vi "Hindbrain Main.vi"(9 "Boat Type":T1(ring), 11 "NotifierReff":T2) -> ()   [LabVIEW 2013]
uses:
  Data/TypeDefs/Notifiers.ctl
  Data/TypeDefs/UTM Location.ctl
  Data/TypeDefs/Sail Set Suggestions.ctl
  Data/TypeDefs/Rudder Set Suggestions.ctl
  <vilib>/myRIO/Common/Instrument Driver Framework/myRIO v1.0/UART/vis/myRIO v1.0 Close UART.vi
  <vilib>/myRIO/Common/Instrument Driver Framework/Utilities/vis/FPGA Ref Manager.vi
  <vilib>/myRIO/Common/Instrument Driver Framework/myRIO v1.0/myRIO v1.0 Reset FPGA.vi
  <vilib>/myRIO/Instrument Drivers/Utilities/Utilities.lvlib
panel:
  in  "XBee Serial Port":refnum<visa-resource-name>
  in  "Queue timeout (ms)":i32=200
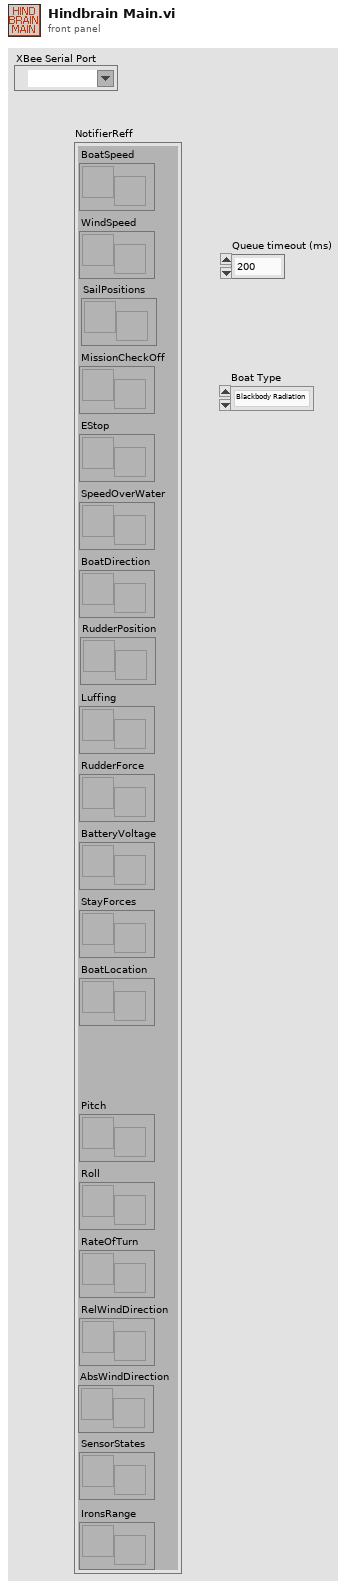
[diagram p1: front panel]
types:
  T1 = enum16{"Blackbody Radiation", "Little boats", "Simulation", "Damn Yankee"}
  T2 = typedef "Notifiers.ctl" = cluster{"BoatSpeed":refnum<notifier>, "WindSpeed":refnum<notifier>, "MissionCheckOff":refnum<notifier>, "EStop":refnum<notifier>, "SpeedOverWater":refnum<notifier>, "BoatDirection":refnum<notifier>, "Luffing":refnum<notifier>, "RudderForce":refnum<notifier>, "BatteryVoltage":refnum<notifier>, "StayForces":refnum<notifier>, "BoatLocation":refnum<notifier>, "Pitch":refnum<notifier>, "Roll":refnum<notifier>, "RateOfTurn":refnum<notifier>, "RelWindDirection":refnum<notifier>, "SailPositions":refnum<notifier>, "RudderPosition":refnum<notifier>, "SensorStates":refnum<notifier>, "IronsRange":refnum<notifier>, "AbsWindDirection":refnum<notifier>}
  T3 = typedef "UTM Location.ctl" = cluster{"UTM Zone":dbl, "Hemisphere":enum16{"North", "South"}, "East":dbl, "North":dbl}
  T4 = typedef "PWM.lvlib/PWM Reference.ctl" = cluster{"myRIO Reference":T5, "PWM Channels Enum":T9, "PWM Configuration":T10}
  T5 = typedef "myRIO Generic Hardware Reference.ctl" = cluster{"myRIO Model":T6, "myRIO Hardware Reference":T7}
  T6 = typedef "Hardware Version Enum.ctl" = enum16{"Unknown", "myRIO-1900", "myRIO-1950"}
  T7 = typedef "myRIO v1.0 Reference.ctl" = cluster{"Generic FPGA Reference":T8, "Allow multiple opens":bool}
  T8 = typedef "Generic FPGA Reference.ctl" = refnum<k20>
  T9 = typedef "PWM Channels Enum.ctl" = enum16{"Not Connected", "C/PWM0", "C/PWM1", "A/PWM0", "A/PWM1", "A/PWM2", "B/PWM0", "B/PWM1", "B/PWM2"}
  T10 = typedef "PWM.lvlib/PWM Configuration.ctl" = cluster{"Frequency":dbl, "Duty Cycle":dbl}
  T11 = cluster{"Airmar VISA Resource":refnum<visa-resource-name>, "Hemisphere VISA Resource":refnum<visa-resource-name>, "Dynamixel VISA Resource":refnum<visa-resource-name>, "Airmar Error":errorcluster, "Hemisphere Error":errorcluster, "Dynamixel Error":errorcluster, "OLD Airmar Refernce Number":refnum<visa-resource-name>, "Rudder PWM Ref":T4, "Rudder Error":errorcluster}
  T12 = typedef "GPS-Compass Queue Cluster.ctl" = cluster{"BoatLocation Queue":refnum<queue>, "BoatDirection Queue":refnum<queue>, "BoatSpeed Queue":refnum<queue>, "RateOfTurn Queue":refnum<queue>, "Pitch Queue":refnum<queue>, "Roll Queue":refnum<queue>}
  T13 = typedef "WindData Queue Cluster.ctl" = cluster{"RelWindDirection Queue":refnum<queue>, "WindSpeed Queue":refnum<queue>, "AbsWindDirection Queue":refnum<queue>}
  T14 = cluster{"Rudder Queue":refnum<queue>, "Shroud Queue":refnum<queue>, "Battery Voltage Queue":refnum<queue>, "Accelerometer Queue":refnum<queue>, "AirmarGPS-Compass Queue Cluster":T12, "Hemisphere Queue Cluster":T12, "Airmar Wind Queue Cluster":T13, "Wind Vane Queue Cluster":T13, "Little Boat Queues":cluster{"Heading Queue":refnum<queue>, "Location Queue":refnum<queue>, "Wind Speed Queue":refnum<queue>, "Tilt Queue":refnum<queue>, "Wind Direction Queue":refnum<queue>}}
  T15 = typedef "Sail Set Suggestions.ctl" = cluster{"MainSailSuggestion":dbl, "JibSailSuggestion":dbl}
  T16 = typedef "Rudder Set Suggestions.ctl" = dbl
  T17 = cluster{"AirmarOnline":bool, "WindvaneOnline":bool, "HemisphereOnline":bool, "RudderForceOnline":bool, "StayForceOnline":bool, "BatteryVoltageOnline":bool, "AccelerometerOnline":bool}
  T18 = cluster{"Nav Data":cluster{"regular expression":string, i32, i32, i32}, "Nav Data":cluster{"regular expression":string, i32, i32, i32}}
  T19 = cluster{"regular expression":string, i32, i32, i32}
  T20 = cluster{"Heading Queue":refnum<queue>, "Location Queue":refnum<queue>, "Wind Speed Queue":refnum<queue>, "Tilt Queue":refnum<queue>, "Wind Direction Queue":refnum<queue>}
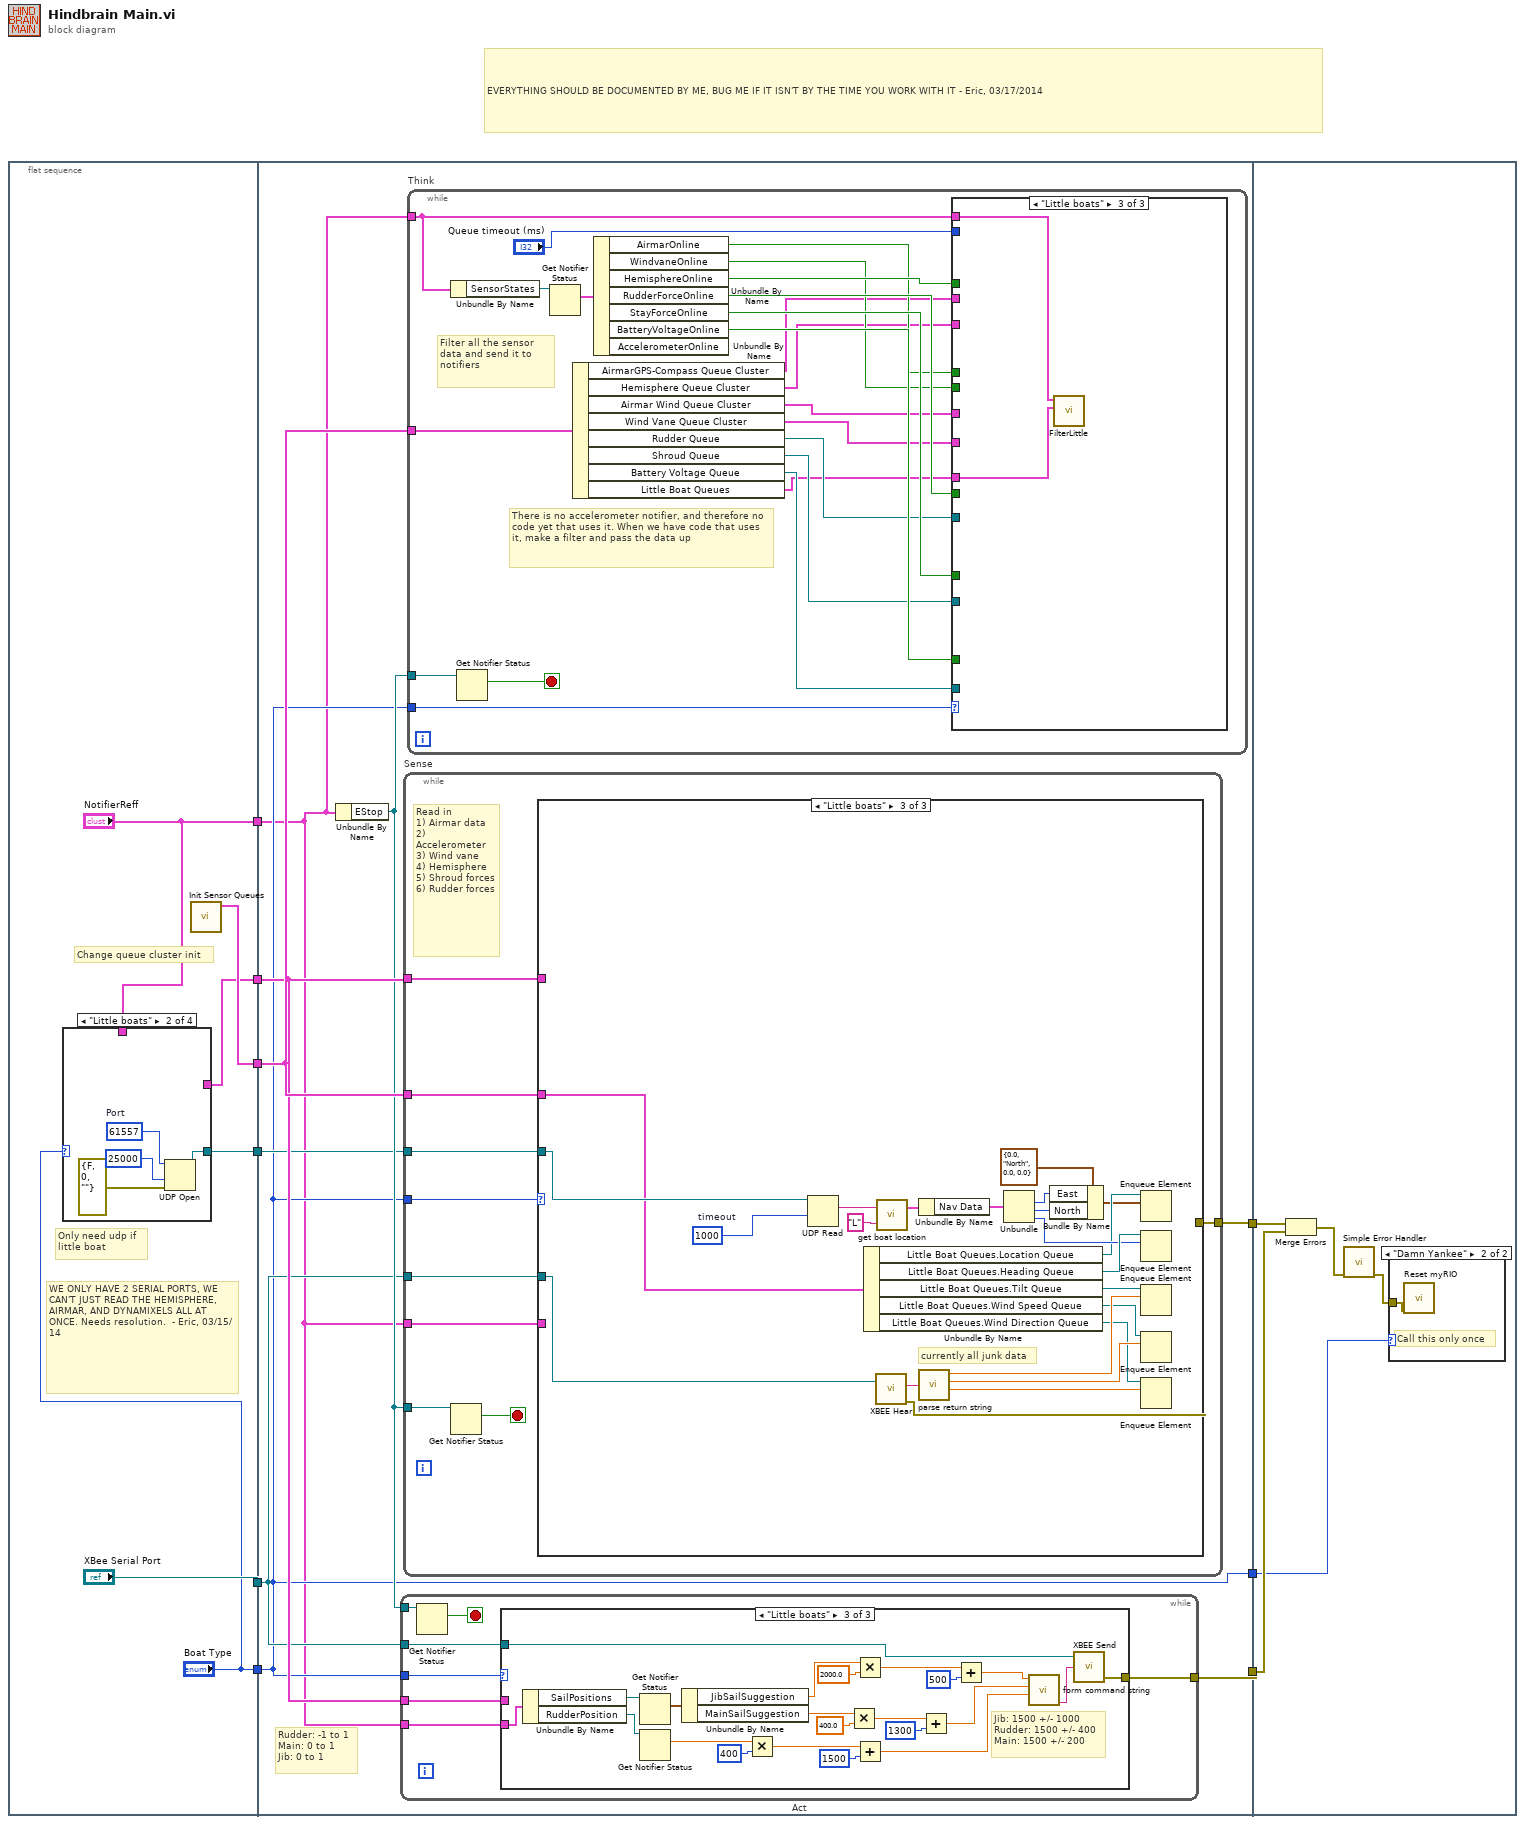
[diagram p0: block diagram]
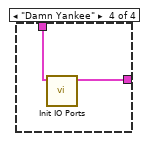
[diagram p4: hidden frame]
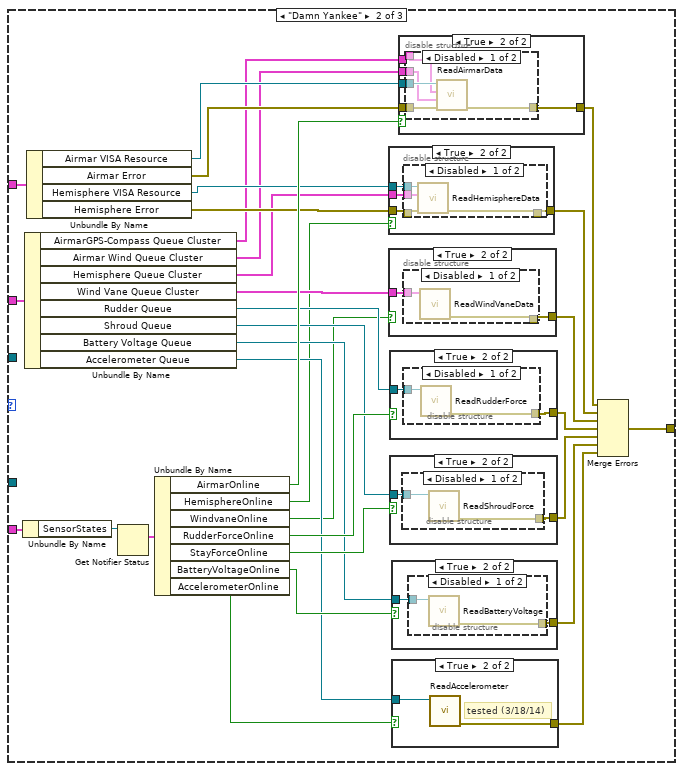
[diagram p6: hidden frame]
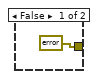
[diagram p7: hidden frame]
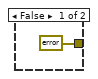
[diagram p8: hidden frame]
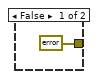
[diagram p10: hidden frame]
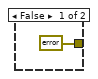
[diagram p12: hidden frame]
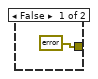
[diagram p14: hidden frame]
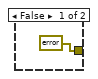
[diagram p16: hidden frame]
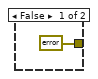
[diagram p18: hidden frame]
diagram:
  # "EVERYTHING SHOULD BE DOCUMENTED BY ME, BUG ME IF IT ISN'T BY THE TIME YOU WORK WITH IT - Eric, 03/17/2014"
  n1 = flat-sequence {
    tunnel: [w15] -> w7
    tunnel: [w11] -> w6
    tunnel: ["Boat Type"] -> w5
    tunnel: ["XBee Serial Port"] -> w4
    tunnel: [w13] -> w3
    tunnel: ["NotifierReff"] -> w1
    tunnel: [w30] -> w9
    tunnel: [w29] -> w8
    tunnel: w7 -> [w28]
    tunnel: w6 -> [w27]
    tunnel: w5 -> [w23]
    tunnel: w4 -> [w25]
    tunnel: w3 -> [w24]
    tunnel: [w23] -> w2
    tunnel: w1 -> [w22]
    tunnel: w9 -> [w255]
    tunnel: w8 -> [w256]
    tunnel: w2 -> [w254]
    frame #0 {
      # "Only need udp if\nlittle boat"
      # "Change queue cluster init"
      # "WE ONLY HAVE 2 SERIAL PORTS, WE CAN'T JUST READ THE HEMISPHERE, AIRMAR, AND DYNAMIXELS ALL AT ONCE. Needs resolution.  - Eric, 03/15/14"
      n2 = case shown="\"Little boats\"" "Boat Type" {
        tunnel: [_ w16 _ _] -> w13
        tunnel: [_ _ _ w21] -> w11
        tunnel: "NotifierReff" -> [_ _ _ w20]
        frame "Blackbody Radiation", Default {
        }
        frame "Little boats" {
          w18 = u16 61557  # Port
          n3 = UDP Open(8:errorcluster {"status"=FALSE, "code"=0, "source"=""} ("error in (no error)"), 9:25000 ("timeout ms (25000)"), 11:w18) -> (port=w16:refnum<k16>)  [unwired: 2 in, 2 out]
        }
        frame "Simulation" {
        }
        frame "Damn Yankee" {
          n4 = call "Init IO Ports.vi"("NotifierReff"=w20) -> ("IO Port Cluster"=w21:T11)  [unwired: 10 in]
        }
      }
      n5 = call "Init Sensor Queues.vi"() -> ("Hindbrain Queue Cluster"=w15:T14)  [unwired: 11 in]
    }
    frame #1 {
      # "Rudder: -1 to 1\nMain: 0 to 1 \nJib: 0 to 1"
      n6 = Unbundle By Name(w22) -> ("EStop"=w26:refnum<notifier>)
      n7 = while "Act" {
        tunnel: w26 -> [w211]
        tunnel: [w210] -> w30
        tunnel: w27 -> [w209]
        tunnel: w23 -> [w208]
        tunnel: w22 -> [w207]
        tunnel: w25 -> [w206]
        stop <- w212 stop-if-true
        n8 = Get Notifier Status(notifier=w211) -> (current notification=w212:bool)  [unwired: 1 in, 4 out]
        n9 = case shown="\"Little boats\"" w208 {
          tunnel: [_ w226 w252] -> w210
          tunnel: w209 -> [_ w224 _]
          tunnel: w207 -> [_ w219 w248]
          tunnel: w206 -> [_ _ w251]
          frame "Blackbody Radiation", Default {
            # "servo + winch"
          }
          frame "Damn Yankee" {
            # "tested (3/18/14)"
            # "Check out what Lindsey was doing with servo/PWM stuff"
            # "Command the two dynamixels and the rudder servo"
            n10 = Unbundle By Name(w224) -> ("Dynamixel VISA Resource"=w223:refnum<visa-resource-name>, "Dynamixel Error"=w222:errorcluster, "Rudder PWM Ref"=w221:T4, "Rudder Error"=w220:errorcluster)
            n11 = Unbundle By Name(w219) -> ("SailPositions"=w218:refnum<notifier>, "RudderPosition"=w217:refnum<notifier>)
            n12 = Get Notifier Status(notifier=w218) -> (current notification=w216:T15, error out=w214:errorcluster)  [unwired: 1 in, 3 out]
            n13 = Get Notifier Status(notifier=w217) -> (current notification=w215:T16, error out=w213:errorcluster)  [unwired: 1 in, 3 out]
            n14 = call "CommandServoPosition.vi"("Error in"=w220, "Suggested Rudder Setpoint"=w215, "PWM Ref In"=w221) -> ("Error out"=w227:errorcluster)  [unwired: 7 in, 1 out]
            n15 = disable-structure shown="Disabled" {
              disable-tunnel: [w231 _] -> w225
              disable-tunnel: w223 -> [w230 _]
              disable-tunnel: w222 -> [w229 _]
              disable-tunnel: w216 -> [w228 _]
              frame Disabled {
                n16 = call "CommandDynamixelPosition.vi"("Error in"=w229, "Sail settings"=w228, "VISA UART port"=w230) -> ("Error out"=w231:errorcluster)  [unwired: 7 in, 1 out]
              }
              frame Enabled {
              }
            }
            n17 = Merge Errors "Merge Errors"(w225, w227, w214, w213) -> (w226:errorcluster)
          }
          frame "Little boats" {
            # "Jib: 1500 +/- 1000\nRudder: 1500 +/- 400\nMain: 1500 +/- 200"
            n18 = Unbundle By Name(w248) -> ("SailPositions"=w250:refnum<notifier>, "RudderPosition"=w249:refnum<notifier>)
            n19 = Get Notifier Status(notifier=w250) -> (current notification=w247:T15)  [unwired: 1 in, 4 out]
            n20 = Get Notifier Status(notifier=w249) -> (current notification=w245:T16)  [unwired: 1 in, 4 out]
            n21 = Unbundle By Name(w247) -> ("JibSailSuggestion"=w239:dbl, "MainSailSuggestion"=w232:dbl)
            n22 = Multiply(x=w245, y=400) -> (x*y=w243:T16)
            n23 = Multiply(x=w232, y=400.0) -> (x*y=w234:dbl)
            n24 = Multiply(x=w239, y=2000.0) -> (x*y=w238:dbl)
            n25 = Add(x=w243, y=1500) -> (x+y=w242:T16)
            n26 = Add(x=w234, y=1300) -> (x+y=w233:dbl)
            n27 = Add(x=w238, y=500) -> (x+y=w237:dbl)
            n28 = call "form command string.vi"("Rudder"=w242, "Main sheet"=w233, "Jib Sheet"=w237) -> ("String"=w253:string)  [unwired: 5 in, 3 out]
            n29 = call "XBEE Send.vi"("String"=w253, "VISA resource name"=w251) -> ("error out"=w252:errorcluster)  [unwired: 1 in, 2 out]
          }
        }
      }
      n30 = while "Sense" {
        tunnel: w22 -> [w35]
        tunnel: [w38] -> w29
        tunnel: w28 -> [w37]
        tunnel: w27 -> [w36]
        tunnel: w26 -> [w34]
        tunnel: w23 -> [w33]
        tunnel: w25 -> [w32]
        tunnel: w24 -> [w31]
        stop <- w39 stop-if-true
        # "Read in\n1) Airmar data\n2) Accelerometer\n3) Wind vane\n4) Hemisphere\n5) Shroud forces\n6) Rudder forces"
        n31 = Get Notifier Status(notifier=w34) -> (current notification=w39:bool)  [unwired: 1 in, 4 out]
        n32 = case shown="\"Little boats\"" w33 {
          tunnel: [_ w71 w136] -> w38
          tunnel: w37 -> [_ w70 w128]
          tunnel: w36 -> [_ w69 _]
          tunnel: w35 -> [_ w40 _]
          tunnel: w32 -> [_ _ w137]
          tunnel: w31 -> [_ _ w134]
          frame "Blackbody Radiation", Default {
          }
          frame "Damn Yankee" {
            n33 = Unbundle By Name(w40) -> ("SensorStates"=w67:refnum<notifier>)
            n34 = Unbundle By Name(w70) -> ("AirmarGPS-Compass Queue Cluster"=w54:T12, "Airmar Wind Queue Cluster"=w53:T13, "Hemisphere Queue Cluster"=w52:T12, "Wind Vane Queue Cluster"=w51:T13, "Rudder Queue"=w60:refnum<queue>, "Shroud Queue"=w58:refnum<queue>, "Battery Voltage Queue"=w56:refnum<queue>, "Accelerometer Queue"=w55:refnum<queue>)
            n35 = Unbundle By Name(w69) -> ("Airmar VISA Resource"=w65:refnum<visa-resource-name>, "Airmar Error"=w64:errorcluster, "Hemisphere VISA Resource"=w63:refnum<visa-resource-name>, "Hemisphere Error"=w62:errorcluster)
            n36 = Get Notifier Status(notifier=w67) -> (current notification=w68:T17)  [unwired: 1 in, 4 out]
            n37 = Unbundle By Name(w68) -> ("AirmarOnline"=w66:bool, "HemisphereOnline"=w49:bool, "WindvaneOnline"=w50:bool, "RudderForceOnline"=w61:bool, "StayForceOnline"=w59:bool, "BatteryVoltageOnline"=w57:bool, "AccelerometerOnline"=w48:bool)
            n38 = case shown="True" w49 {
              tunnel: [errorcluster {"status"=FALSE, "code"=0, "source"=""} ("Error out") w94] -> w42
              tunnel: w63 -> [_ w93]
              tunnel: w62 -> [_ w92]
              tunnel: w52 -> [_ w91]
              frame False {
              }
              frame True {
                n39 = disable-structure shown="Disabled" {
                  disable-tunnel: [w98 _] -> w94
                  disable-tunnel: w93 -> [w97 _]
                  disable-tunnel: w92 -> [w96 _]
                  disable-tunnel: w91 -> [w95 _]
                  frame Disabled {
                    n40 = call "ReadHemisphereData.vi"("Error in"=w96, "Hemisphere Queue Cluster"=w95, "VISA UART port"=w97) -> ("Error out"=w98:errorcluster)  [unwired: 8 in]
                  }
                  frame Enabled {
                  }
                }
              }
            }
            n41 = case shown="True" w50 {
              tunnel: [errorcluster {"status"=FALSE, "code"=0, "source"=""} ("error out") w101] -> w43
              tunnel: w51 -> [_ w100]
              frame False {
              }
              frame True {
                n42 = disable-structure shown="Disabled" {
                  disable-tunnel: [w103 _] -> w101
                  disable-tunnel: w100 -> [w102 _]
                  frame Disabled {
                    n43 = call "ReadWindVaneData.vi"("Wind Vane Queue Cluster"=w102) -> ("error out"=w103:errorcluster)  [unwired: 9 in, 1 out]
                  }
                  frame Enabled {
                  }
                }
              }
            }
            n44 = case shown="True" w61 {
              tunnel: [errorcluster {"status"=FALSE, "code"=0, "source"=""} ("error out") w87] -> w44
              tunnel: w60 -> [_ w86]
              frame False {
              }
              frame True {
                n45 = disable-structure shown="Disabled" {
                  disable-tunnel: [w89 _] -> w87
                  disable-tunnel: w86 -> [w88 _]
                  frame Disabled {
                    n46 = call "ReadRudderForce.vi"("Queue in"=w88) -> ("error out"=w89:errorcluster)  [unwired: 10 in]
                  }
                  frame Enabled {
                  }
                }
              }
            }
            n47 = case shown="True" w59 {
              tunnel: w58 -> [_ w82]
              tunnel: [errorcluster {"status"=FALSE, "code"=0, "source"=""} ("error out") w81] -> w45
              frame False {
              }
              frame True {
                n48 = disable-structure shown="Disabled" {
                  disable-tunnel: w82 -> [w84 _]
                  disable-tunnel: [w83 _] -> w81
                  frame Disabled {
                    n49 = call "ReadShroudForce.vi"("Queue in"=w84) -> ("error out"=w83:errorcluster)  [unwired: 9 in, 1 out]
                  }
                  frame Enabled {
                  }
                }
              }
            }
            n50 = case shown="True" w57 {
              tunnel: w56 -> [_ w77]
              tunnel: [errorcluster {"status"=FALSE, "code"=0, "source"=""} ("error out") w76] -> w46
              frame False {
              }
              frame True {
                n51 = disable-structure shown="Disabled" {
                  disable-tunnel: w77 -> [w79 _]
                  disable-tunnel: [w78 _] -> w76
                  frame Disabled {
                    n52 = call "ReadBatteryVoltage.vi"("Queue in"=w79) -> ("error out"=w78:errorcluster)  [unwired: 9 in, 1 out]
                  }
                  frame Enabled {
                  }
                }
              }
            }
            n53 = case shown="True" w48 {
              tunnel: [errorcluster {"status"=FALSE, "code"=0, "source"=""} ("error out") w74] -> w47
              tunnel: w55 -> [_ w73]
              frame False {
              }
              frame True {
                # "tested (3/18/14)"
                n54 = call "ReadAccelerometer.vi"("Accelerometer Queue"=w73) -> ("error out"=w74:errorcluster)  [unwired: 10 in]
              }
            }
            n55 = case shown="True" w66 {
              tunnel: w65 -> [_ w109]
              tunnel: w54 -> [_ w106]
              tunnel: w64 -> [_ w108]
              tunnel: [errorcluster {"status"=FALSE, "code"=0, "source"=""} ("Error out") w107] -> w41
              tunnel: w53 -> [_ w105]
              frame False {
              }
              frame True {
                n56 = disable-structure shown="Disabled" {
                  disable-tunnel: w109 -> [w114 _]
                  disable-tunnel: w108 -> [w113 _]
                  disable-tunnel: [w112 _] -> w107
                  disable-tunnel: w106 -> [w111 _]
                  disable-tunnel: w105 -> [w110 _]
                  frame Disabled {
                    n57 = call "ReadAirmarData.vi"("Error in"=w113, "Airmar Wind Queue Cluster"=w110, "AirmarGPS-Compass Queue Cluster"=w111, "VISA UART port"=w114) -> ("Error out"=w112:errorcluster)  [unwired: 7 in]
                  }
                  frame Enabled {
                  }
                }
              }
            }
            n58 = Merge Errors "Merge Errors"(w41, w42, w43, w44, w45, w46, w47) -> (w71:errorcluster)
          }
          frame "Little boats" {
            w133 = 1000  # timeout
            # "currently all junk data"
            n59 = UDP Read(connection ID=w134, timeout ms (25000)=w133) -> (data out=w132:string)  [unwired: 2 in, 4 out]
            n60 = Unbundle By Name(w128) -> ("Little Boat Queues.Location Queue"=w122:refnum<queue>, "Little Boat Queues.Heading Queue"=w124:refnum<queue>, "Little Boat Queues.Tilt Queue"=w120:refnum<queue>, "Little Boat Queues.Wind Speed Queue"=w118:refnum<queue>, "Little Boat Queues.Wind Direction Queue"=w116:refnum<queue>)
            n61 = call "XBEE Hear.vi"("VISA resource name"=w137) -> ("String Received"=w135:string, "error out"=w136:errorcluster)  [unwired: 1 in, 2 out]
            n62 = call "get boat location.vi"("Tug"="L", "Nav String"=w132) -> ("Tug Nav Data"=w130:T18)  [unwired: 1 out]
            n63 = Unbundle By Name(w130) -> ("Nav Data"=w129:T19)
            n64 = call "parse return string.vi"("Return String"=w135) -> ("Tilt"=w119:dbl, "Wind Speed"=w117:dbl, "Wind Direction"=w115:dbl)  [unwired: 1 out]
            n65 = Unbundle(w129) -> (w126:i32, w125:i32, w123:i32)  [unwired: 1 out]
            n66 = Bundle By Name(cluster=T3 {"UTM Zone"=0.0, "Hemisphere"=enum."North", "East"=0.0, "North"=0.0} ("UTM Location"), "East"=w126, "North"=w125) -> (w121:T3)
            n67 = Enqueue Element(queue=w122, element=w121) -> ()  [unwired: 2 in, 3 out]
            n68 = Enqueue Element(queue=w124, element=w123) -> ()  [unwired: 2 in, 3 out]
            n69 = Enqueue Element(queue=w120, element=w119) -> ()  [unwired: 2 in, 3 out]
            n70 = Enqueue Element(queue=w118, element=w117) -> ()  [unwired: 2 in, 3 out]
            n71 = Enqueue Element(queue=w116, element=w115) -> ()  [unwired: 2 in, 3 out]
          }
        }
      }
      n72 = while "Think" {
        tunnel: w26 -> [w158]
        tunnel: w28 -> [w157]
        tunnel: w22 -> [w143]
        tunnel: w23 -> [w141]
        stop <- w159 stop-if-true
        # "There is no accelerometer notifier, and therefore no code yet that uses it. When we have code that uses it, make a filter and pass the data up"
        # "Filter all the sensor data and send it to notifiers"
        n73 = Unbundle By Name(w143) -> ("SensorStates"=w144:refnum<notifier>)
        n74 = Get Notifier Status(notifier=w158) -> (current notification=w159:bool)  [unwired: 1 in, 4 out]
        n75 = Get Notifier Status(notifier=w144) -> (current notification=w156:T17)  [unwired: 1 in, 4 out]
        n76 = Unbundle By Name(w157) -> ("AirmarGPS-Compass Queue Cluster"=w145:T12, "Hemisphere Queue Cluster"=w139:T12, "Airmar Wind Queue Cluster"=w138:T13, "Wind Vane Queue Cluster"=w146:T13, "Rudder Queue"=w147:refnum<queue>, "Shroud Queue"=w148:refnum<queue>, "Battery Voltage Queue"=w149:refnum<queue>, "Little Boat Queues"=w140:T20)
        n77 = Unbundle By Name(w156) -> ("AirmarOnline"=w151:bool, "WindvaneOnline"=w150:bool, "HemisphereOnline"=w152:bool, "RudderForceOnline"=w155:bool, "StayForceOnline"=w154:bool, "BatteryVoltageOnline"=w153:bool)  [unwired: 1 out]
        n78 = case shown="\"Little boats\"" w141 {
          tunnel: w155 -> [_ w174 _]
          tunnel: w154 -> [_ w173 _]
          tunnel: w153 -> [_ w172 _]
          tunnel: w152 -> [_ w171 _]
          tunnel: w151 -> [_ w170 _]
          tunnel: w150 -> [_ w169 _]
          tunnel: w149 -> [_ w168 _]
          tunnel: w148 -> [_ w167 _]
          tunnel: w147 -> [_ w166 _]
          tunnel: w146 -> [_ w165 _]
          tunnel: w138 -> [_ w164 _]
          tunnel: w145 -> [_ w163 _]
          tunnel: w139 -> [_ w162 _]
          tunnel: w143 -> [_ w161 w205]
          tunnel: "Queue timeout (ms)" -> [_ w160 _]
          tunnel: w140 -> [_ _ w204]
          frame "Blackbody Radiation", Default {
          }
          frame "Damn Yankee" {
            n79 = case shown="False" w171 {
              tunnel: w170 -> [w188 _]
              tunnel: w161 -> [w186 w193]
              tunnel: w163 -> [w187 _]
              tunnel: w162 -> [_ w194]
              tunnel: w160 -> [w185 w192]
              frame False {
                n80 = case shown="True" w188 {
                  tunnel: w187 -> [_ w191]
                  tunnel: w186 -> [_ w190]
                  tunnel: w185 -> [_ w189]
                  frame False {
                  }
                  frame True {
                    n81 = call "FilterAirmarGPS.vi"("Queue timeout (ms)"=w189, "NotifierReff"=w190, "AirmarGPS-Compass Queue Cluster"=w191) -> ()  [unwired: 9 in]
                  }
                }
              }
              frame True {
                n82 = call "FilterHemisphere.vi"("Queue timeout (ms)"=w192, "NotifierReff"=w193, "Hemisphere Queue Cluster"=w194) -> ()  [unwired: 9 in]
              }
            }
            n83 = case shown="False" w170 {
              tunnel: w169 -> [w178 _]
              tunnel: w165 -> [w177 _]
              tunnel: w164 -> [_ w184]
              tunnel: w161 -> [w176 w183]
              tunnel: w160 -> [w175 w182]
              frame False {
                n84 = case shown="True" w178 {
                  tunnel: w177 -> [_ w181]
                  tunnel: w176 -> [_ w180]
                  tunnel: w175 -> [_ w179]
                  frame False {
                  }
                  frame True {
                    n85 = call "FilterWindVane.vi"("Queue timeout (ms)"=w179, "NotifierReff 2"=w180, "Wind Vane Queue Cluster"=w181) -> ()  [unwired: 9 in]
                  }
                }
              }
              frame True {
                n86 = call "FilterAirmarWind.vi"("Queue timeout (ms)"=w182, "NotifierReff"=w183, "Airmar Wind Queue Cluster"=w184) -> ()  [unwired: 9 in]
              }
            }
            n87 = case shown="True" w174 {
              tunnel: w166 -> [_ w203]
              tunnel: w161 -> [_ w202]
              tunnel: w160 -> [_ w201]
              frame False {
              }
              frame True {
                n88 = call "FilterRudder.vi"("Queue timeout (ms)"=w201, "NotifierReff 2"=w202, "Queue in"=w203) -> ()  [unwired: 9 in]
              }
            }
            n89 = case shown="True" w173 {
              tunnel: w167 -> [_ w200]
              tunnel: w161 -> [_ w199]
              tunnel: w160 -> [_ w198]
              frame False {
              }
              frame True {
                n90 = call "FilterShrouds.vi"("Queue timeout (ms)"=w198, "NotifierReff 2"=w199, "Queue in"=w200) -> ()  [unwired: 9 in]
              }
            }
            n91 = case shown="True" w172 {
              tunnel: w168 -> [_ w197]
              tunnel: w161 -> [_ w196]
              tunnel: w160 -> [_ w195]
              frame False {
              }
              frame True {
                n92 = call "FilterBatteryVoltage.vi"("Queue timeout (ms)"=w195, "NotifierReff"=w196, "Queue in"=w197) -> ()  [unwired: 9 in]
              }
            }
          }
          frame "Little boats" {
            n93 = call "FilterLittle.vi"("Little Boat Queues"=w204, "NotifierReff"=w205) -> ()  [unwired: 10 in]
          }
        }
      }
    }
    frame #2 {
      n94 = Merge Errors "Merge Errors"(w256, w255) -> (w258:errorcluster)
      n95 = call <vilib>:"Simple Error Handler.vi"("error in (no error)"=w258) -> ("error out"=w257:errorcluster)  [unwired: 4 in, 4 out]
      n96 = case shown="\"Damn Yankee\"" w254 {
        tunnel: w257 -> [_ w259]
        frame "Blackbody Radiation", Default {
        }
        frame "Damn Yankee" {
          # "Call this only once"
          n97 = call <vilib>:"Reset myRIO.vi"("error in (no error)"=w259) -> ()  [unwired: 10 in, 1 out]
        }
      }
    }
  }
